vi "Open.vi"(8 "error in (no error)":errorcluster, 10 "Interface_type":T1="DALI", 11 "Dali_usb_tridonics in":refnum<class "Dali_usb_tridonics.lvclass">) -> (0 "error out":errorcluster, 3 "Dali_usb_tridonics out":refnum<class "Dali_usb_tridonics.lvclass">)   [LabVIEW 2014, in "Driver_interaction.lvlib" / "Dali_usb_tridonics.lvclass"]
uses:
  Dali_usb_tridonics.lvclass
  _Driver_interaction/Controls/Interface_type.ctl
  Dali_usb_tridonics.lvclass/Dali_usb_tridonics.ctl
  _Driver_interaction/_Driver_interaction.lvclass
  Vendor/Dali_usb.lvlib
panel:
  out "device_handle":i32
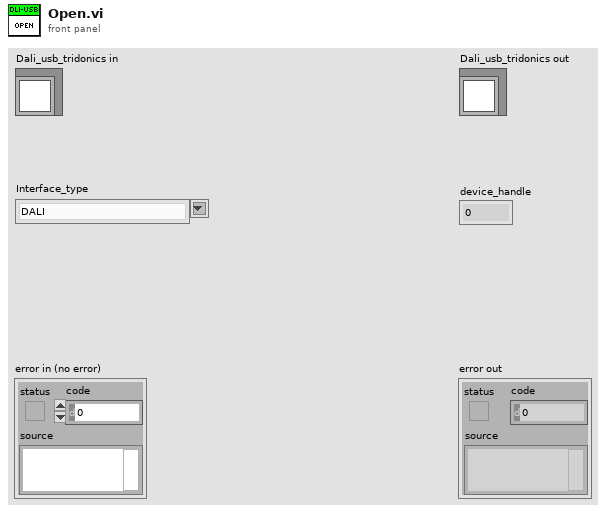
[diagram p1: front panel]
types:
  T1 = typedef "Driver_interaction.lvlib/_Driver_interaction.lvclass/Interface_type.ctl" = string
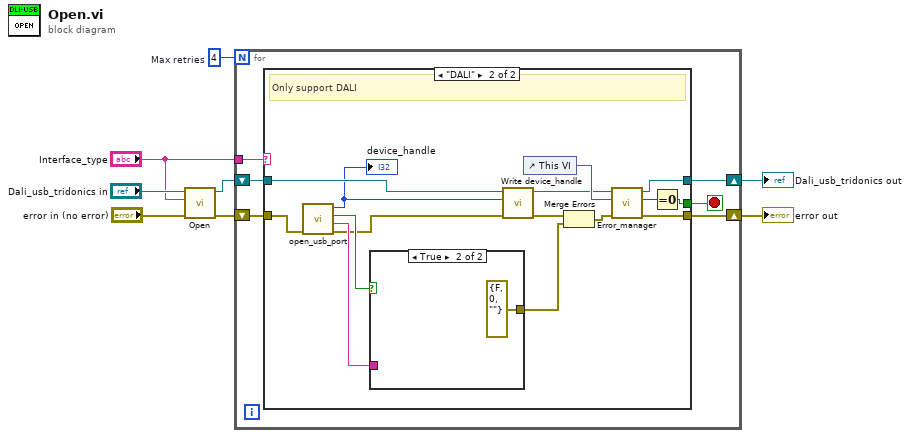
[diagram p0: block diagram]
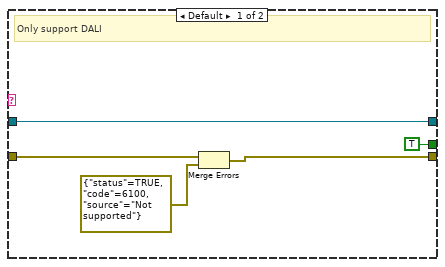
[diagram p2: hidden frame]
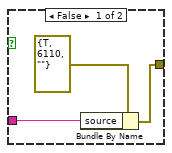
[diagram p3: hidden frame]
diagram:
  w1 = 4  # Max retries
  n1 = call-parent "Open.vi"("error in (no error)"="error in (no error)", "Interface_type"="Interface_type", "_Driver_interaction in"="Dali_usb_tridonics in") -> ("error out"=w4:errorcluster, "_Driver_interaction out"=w3:refnum<class "Dali_usb_tridonics.lvclass">)  [unwired: 7 in]
  n2 = for {
    N: w1 -> [_]
    tunnel: "Interface_type" -> [w14]
    shift-right: [w13] -> w5
    shift-left: w4 -> [w12]
    shift-right: [w10] -> w2
    shift-left: w3 -> [w11]
    stop <- w9 stop-if-true
    n3 = case shown="\"DALI\"" w14 {
      tunnel: [w16 w25] -> w13
      tunnel: w12 -> [w18 w34]
      tunnel: w11 -> [w19 w30]
      tunnel: [w19 w20] -> w10
      tunnel: [TRUE w22] -> w9
      frame Default {
        # "Only support DALI"
        n4 = Merge Errors(w18, errorcluster {"status"=TRUE, "code"=6100, "source"="Not supported"} ("error out")) -> (w16:errorcluster)
      }
      frame "DALI" {
        # "Only support DALI"
        n5 = call "open_usb_port.vi"("error in (no error)"=w34) -> ("error out"=w29:errorcluster, "failstring"=w32:string, "opened"=w33:bool, "device_handle"=w27:i32)  [unwired: 7 in]
        "device_handle" <- w27
        n6 = case shown="True" w33 {
          tunnel: w32 -> [w36 _]
          tunnel: [w35 errorcluster {"status"=FALSE, "code"=0, "source"=""} ("error out")] -> w31
          frame False {
            n7 = Bundle By Name(cluster=errorcluster {"status"=TRUE, "code"=6110, "source"=""} ("error out"), "source"=w36) -> (w35:errorcluster)
          }
          frame True {
          }
        }
        n8 = call "Write device_handle.vi"("error in (no error)"=w29, "device_handle"=w27, "Dali_usb_tridonics in"=w30) -> ("error out"=w28:errorcluster, "Dali_usb_tridonics out"=w21:refnum<class "Dali_usb_tridonics.lvclass">)  [unwired: 7 in]
        n9 = control-ref of="This VI"() -> (w24:refnum<vi>)
        n10 = Merge Errors(w28, w31) -> (w26:errorcluster)
        n11 = call-dynamic "Error_manager.vi"("error in (no error)"=w26, "Caller VI"=w24, "Dali_usb_tridonics in"=w21) -> ("error out"=w25:errorcluster, "code"=w23:i32, "Dali_usb_tridonics out"=w20:refnum<class "Dali_usb_tridonics.lvclass">)  [unwired: 4 in, 2 out]
        n12 = Equal To 0?(x=w23) -> (x = 0?=w22:bool)
      }
    }
  }
  "error out" <- w5
  "Dali_usb_tridonics out" <- w2
